vi "MotorDeadband.vi"(9 "DBPercent":dbl, 11 "MotorIn":u16) -> (3 "MotorOut":u16)   [LabVIEW 2013, in "ProcessorHelperFunctions.lvlib"]
uses:
  ProcessorHelperFunctions.lvlib
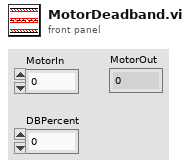
[diagram p1: front panel]
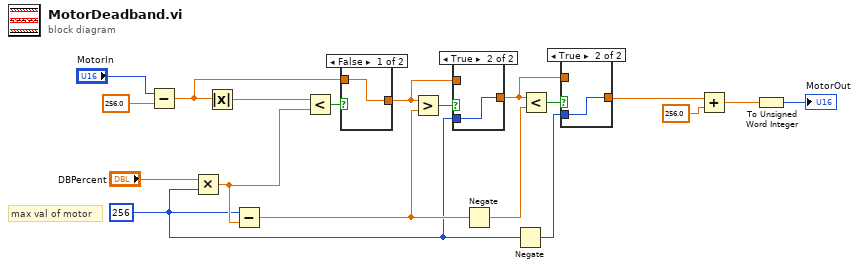
[diagram p0: block diagram]
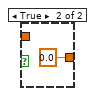
[diagram p4: hidden frame]
diagram:
  w8 = 256
  # "max val of motor"
  n1 = Subtract(x="MotorIn", y=256.0 ("x")) -> (x-y=w4:dbl)
  n2 = Multiply(x="DBPercent", y=w8) -> (x*y=w10:dbl)
  n3 = Absolute Value(x=w4) -> (abs(x)=w13:dbl)
  n4 = Subtract(x=w8, y=w10) -> (x-y=w9:dbl)
  n5 = Less?(x=w13, y=w10) -> (x < y?=w18:bool)
  n6 = case shown="False" w18 {
    tunnel: w4 -> [w20 _]
    tunnel: [w20 0.0 ("JoystickIn[0]")] -> w16
    frame False {
    }
    frame True {
    }
  }
  n7 = Greater?(x=w16, y=w9) -> (0:w17:bool)
  n8 = case shown="True" w17 {
    tunnel: [w22 w23] -> w14
    tunnel: w16 -> [w22 _]
    tunnel: w8 -> [_ w23]
    frame False {
    }
    frame True {
    }
  }
  n9 = Negate(x=w9) -> (-x=w7:dbl)
  n10 = Negate(x=w8) -> (-x=w6:i32)
  n11 = Less?(x=w14, y=w7) -> (x < y?=w15:bool)
  n12 = case shown="True" w15 {
    tunnel: [w24 w25] -> w2
    tunnel: w14 -> [w24 _]
    tunnel: w6 -> [_ w25]
    frame False {
    }
    frame True {
    }
  }
  n13 = Add(x=w2, y=256.0) -> (x+y=w1:dbl)
  n14 = To Unsigned Word Integer(number=w1) -> (unsigned 16bit integer=→"MotorOut":u16)
